vi "Get Intensity Graph Y Scale.vi"(8 "error in (no error)":errorcluster, 11 "graph_utilities in":refnum<class "graph_utilities.lvclass">) -> (0 "error out":errorcluster, 1 "Y Scale.Offset and Multiplier":T1, 2 "Y Scale":dbl[](array[numeric]), 3 "graph_utilities out":refnum<class "graph_utilities.lvclass">)   [LabVIEW 2019, in "graph_utilities.lvclass"]
doc: "Get the Y Scale of the Intensity Graph (Both Y Array and Y Offset and Multiplier)"
uses:
  graph_utilities.lvclass
  <vilib>/Utility/miscctls.llb/LVOffsetAndMultiplierTypeDef.ctl
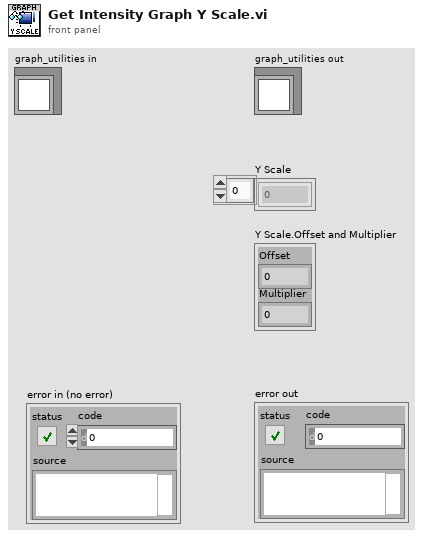
[diagram p1: front panel]
types:
  T1 = typedef "LVOffsetAndMultiplierTypeDef.ctl" = cluster{"Offset":dbl, "Multiplier":dbl}
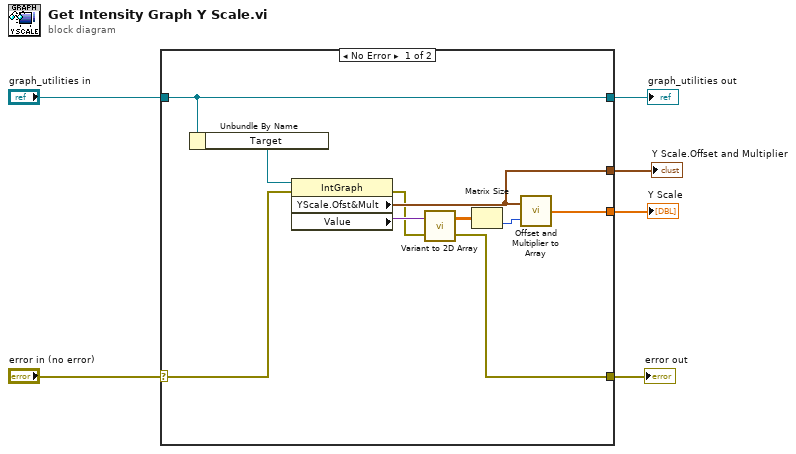
[diagram p0: block diagram]
diagram:
  n1 = case shown="No Error" "error in (no error)" {
    selector: "error in (no error)" -> [w16 w18]
    tunnel: [w7 w18] -> w6
    tunnel: "graph_utilities in" -> [w15 w17]
    tunnel: [w15 w17] -> w3
    tunnel: [w14 _] -> w2
    tunnel: [w12 _] -> w1
    frame No Error {
      n2 = Unbundle By Name(w15) -> ("Target"=w11:refnum<vi>)
      n3 = property on="Property Node" class="IntGraph"(reference=w11, error in=w16) -> (error out=w8:errorcluster, "YScale.Ofst&Mult"=w12:T1, "Value"=w10:variant)  [unwired: 1 out]
      n4 = call "Variant to 2D Array.vi"("error in (no error)"=w8, "Value"=w10) -> ("error out"=w7:errorcluster, "Array"=w9:dbl[][])
      n5 = Matrix Size(0:w9) -> (2:w13:i32)  [unwired: 1 out]
      n6 = call "Offset and Multiplier to Array.vi"("Size"=w13, "Offset and Multiplier"=w12) -> ("Array"=w14:dbl[])
    }
    frame Error {
    }
  }
  "Y Scale" <- w2
  "error out" <- w6
  "graph_utilities out" <- w3
  "Y Scale.Offset and Multiplier" <- w1
